vi "manual_display.vi"() -> ()   [LabVIEW 2020]
uses:
  <vilib>/Analysis/1siggen.llb/Ramp Pattern by Samples.vi
  <vilib>/Waveform/WDTOps.llb/WDT Get Waveform Subset DBL.vi
  <vilib>/Analysis/1siggen.llb/Ramp Pattern by Delta.vi
  <vilib>/Analysis/NI_AALBase.lvlib
  <vilib>/Analysis/NI_AALPro.lvlib
panel:
  out "gps-es sebesség\ngrafikon":cluster{timestamp[], "Y":dbl[]}[](graph)
  in  "másolás mód":bool
  in  "gps elcsúsztatás [s]":dbl format="%#_13g"
  out "elemzõ grafikon":T1(graph)
  in  "high cutoff freq":dbl=10.0 format="%#_13g"
  in  "low cutoff freq":dbl=0.05 format="%#_13g"
  out "impulse szum/mean\n(összes csapás az átlagos \ncsapásszámon)":dbl format="%0.2f"
  out "inspected resultant":waveform(dbl)(graph)
  out "Z axis SNR mean":dbl format="%0.2f"
  out "Z axis SNR standard deviation":dbl format="%0.2f"
  out "resultant SNR mean":dbl format="%0.2f"
  out "resultant SNR standard deviation":dbl format="%0.2f"
  out "Y axis SNR mean":dbl format="%0.2f"
  out "Y axis SNR standard deviation":dbl format="%0.2f"
  out "X axis SNR standard deviation":dbl format="%0.2f"
  out "X axis SNR mean":dbl format="%0.2f"
  out "impulse mean":dbl format="%0.2f"
  out "Z axis SNR":cluster{"Ramp Pattern":dbl[], dbl[]}[](graph)
  out "Y axis SNR":cluster{"Ramp Pattern":dbl[], dbl[]}[](graph)
  out "X axis SNR":cluster{"Ramp Pattern":dbl[], dbl[]}[](graph)
  out "resultant SNR":cluster{"Ramp Pattern":dbl[], dbl[]}[](graph)
  in  "felharmonikus N":i32=3
  out "standard deviation of peaks":dbl format="%0.2f"
  out "SNR":dbl
  in  "SNR window width [Hz]":dbl=0.2
  out "impulse  szum":dbl format="%0.2f"
  out "impulse standard deviation":dbl format="%0.2f"
  in  "invert":bool
  out "csapás impulzus":cluster{"Ramp Pattern":dbl[], dbl[]}(graph)
  in  "peak detect width":i32=5 min=3
  in  "avg window size":i32=5
  in  "threshold":dbl=0.25 format="%0.2f"
  out "mean of peaks":dbl format="%0.2f"
  out "csapásszám":cluster{"Ramp Pattern":dbl[], dbl[]}[](graph)
  in  "felbontás [s]":dbl=20.0
  out "Átlag Csapásszám [stroke/m]":dbl
  out "PSD":cluster{"f0":dbl, "df":dbl, "magnitude":dbl[]}[](graph)
  in  "crossing level":dbl
  in  "Cursor reset":bool=TRUE
  out "inspection":cluster{"Y":dbl[], "Y":dbl[]}[](graph)
  in  "Sec":dbl=60.0
  in  "Start Cursor":timestamp
  in  "inspect":bool
  in  "path to binary file":path=path "C:/Users/Lenovo/Desktop/canoe_akti_data"
  in  "stop":bool
  out "inspected section":waveform(dbl)[](graph)
  out "read in data":waveform(dbl)[](graph)
  # "[felbontas]mp-es ablakokkal számított SNR meta adatok"
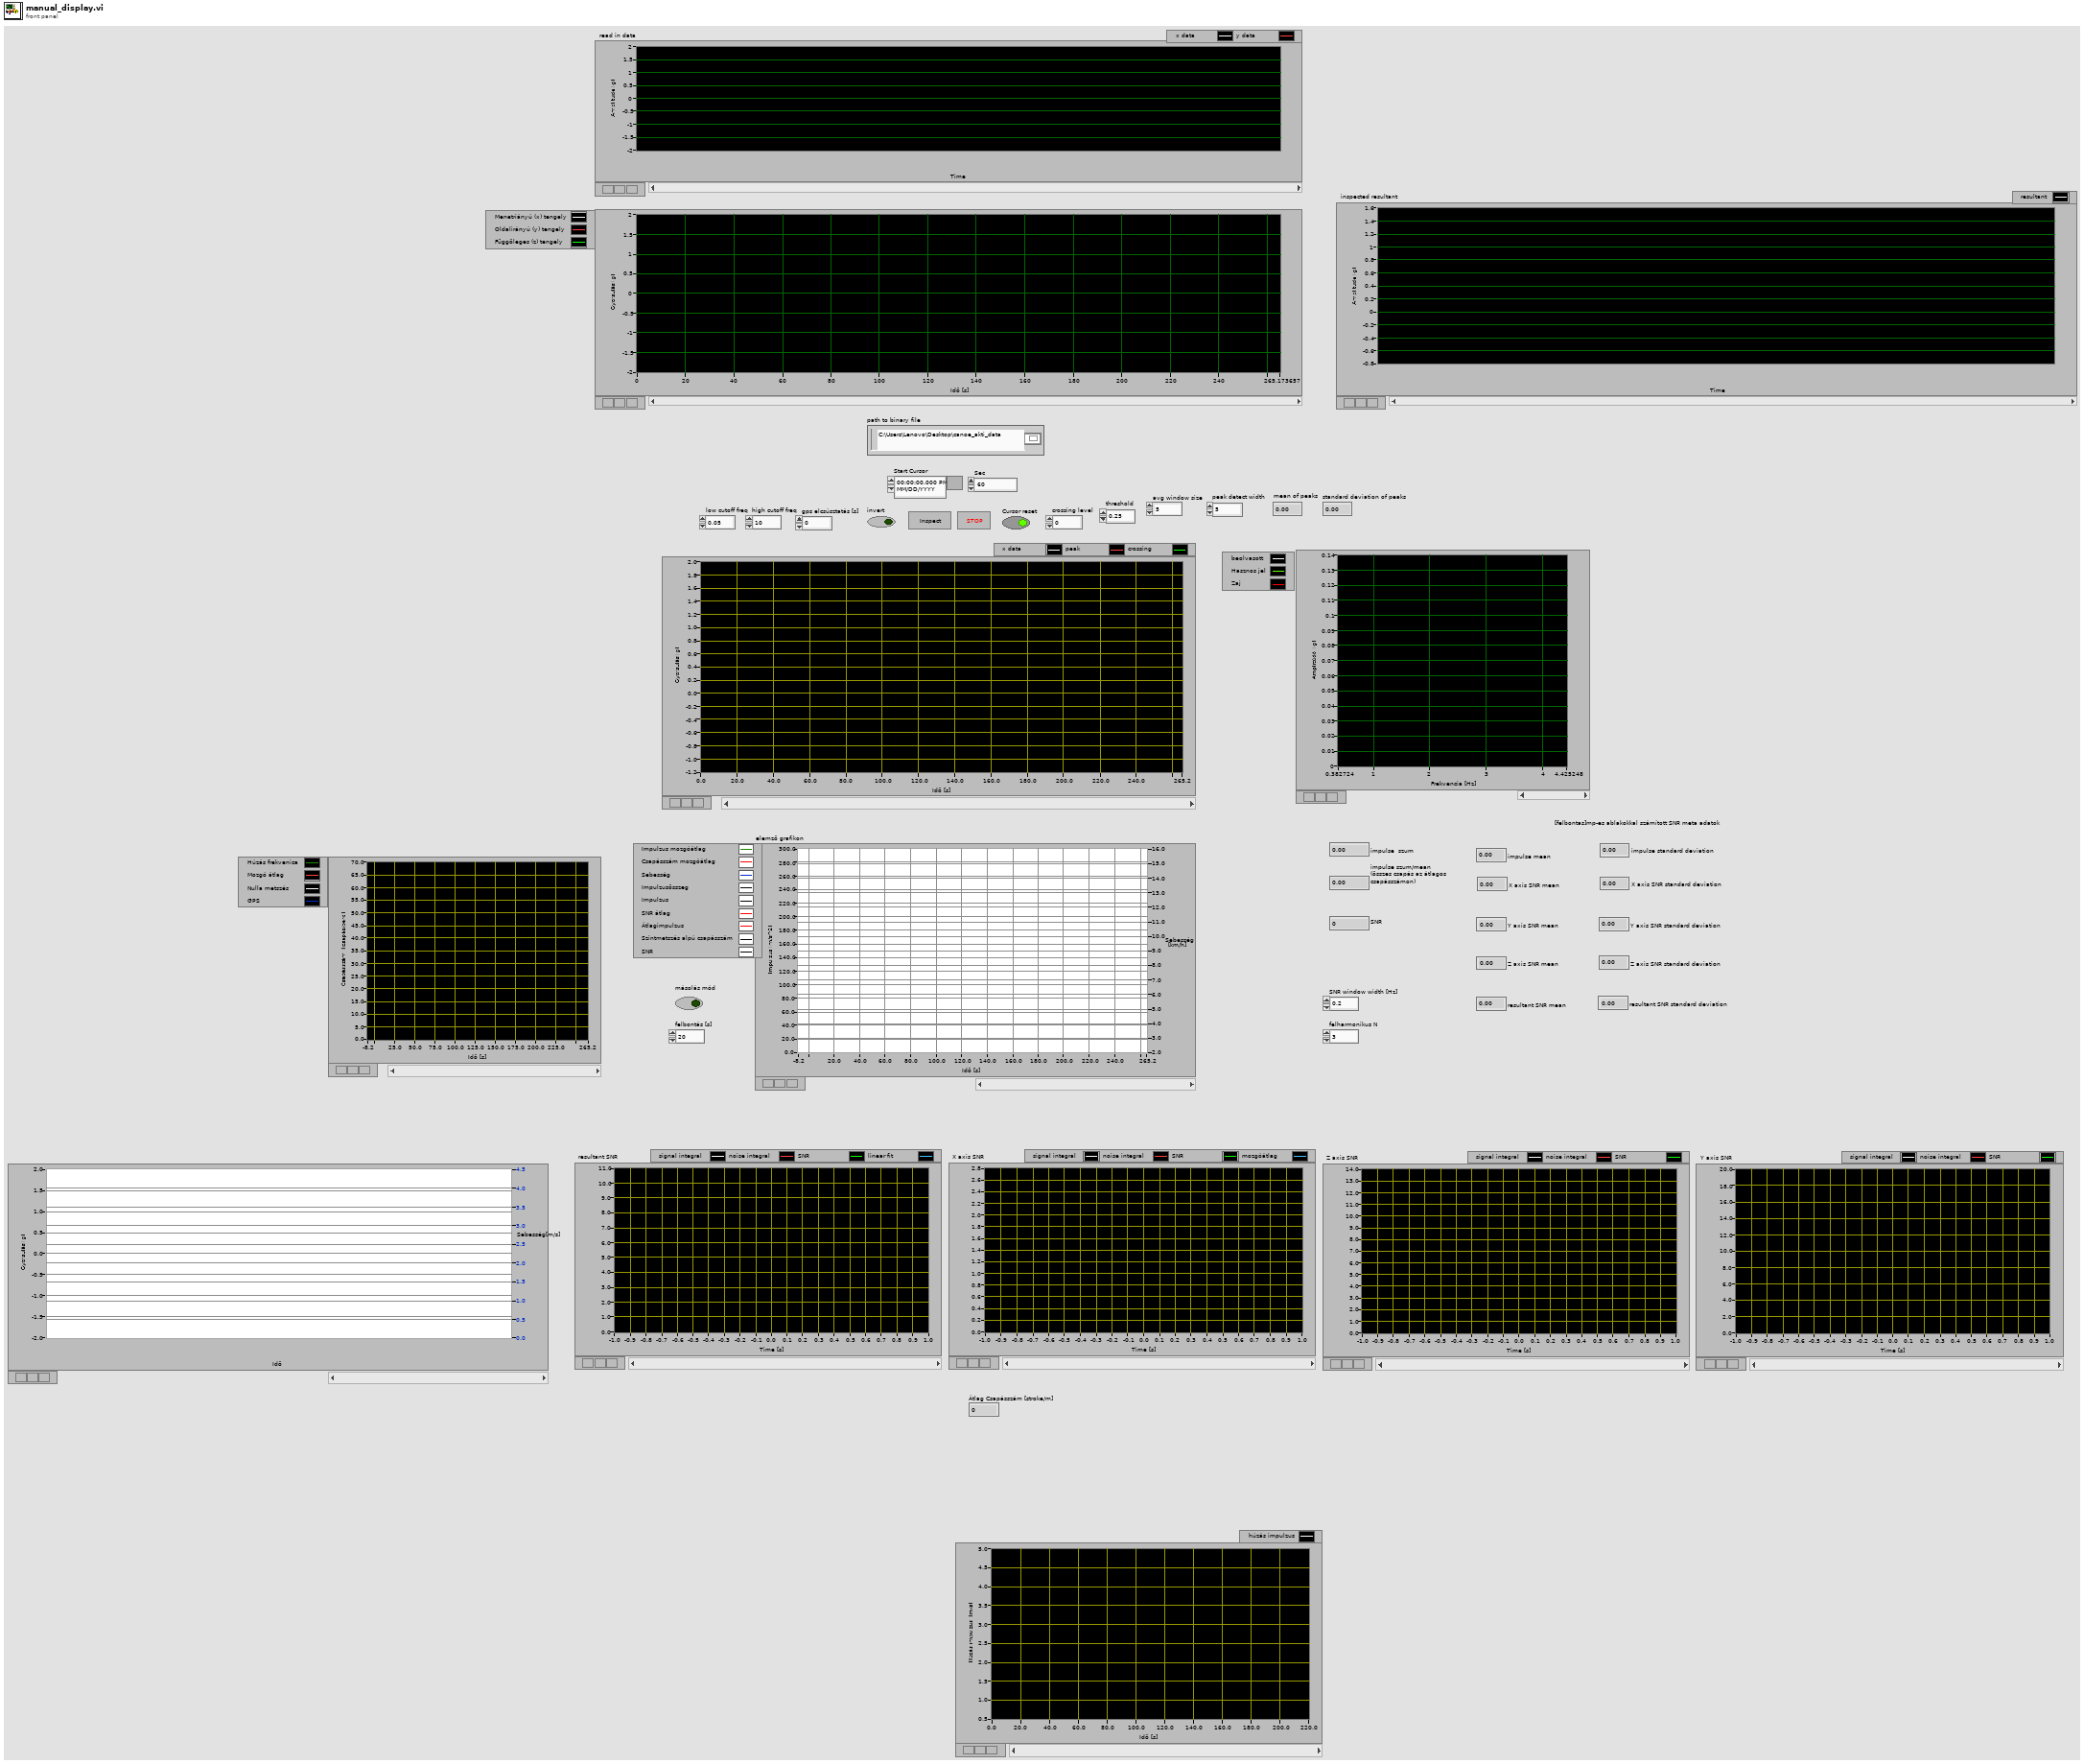
[diagram p1: front panel]
types:
  T1 = cluster{"Ramp Pattern":dbl[], "averaged X":dbl[]}[]
  T2 = typedef "control_all_in_one_package.ctl" = cluster{"memory structure":T3, "actigraph settings":T4, "time informations":T5, "measurement data":T6}
  T3 = typedef "control_memory_structure.ctl" = cluster{"length of metadata [byte]":i32, "length of page [byte]":i32, "length of measurement data on page [byte]":i32, "length of dataset [byte]":i32}
  T4 = typedef "control_measurement_settings.ctl" = cluster{"sampling frequency [Hz]":dbl, "measurement interval [± g]":i32, "high precision?":bool, "number of pages":i32, "rate code":i32, "range code":i32, "id":i32}
  T5 = typedef "control_time_informations.ctl" = cluster{"starting time":timestamp, "ending time":timestamp, "dt[s]":dbl, "sampling rate [Hz]":dbl, "length":dbl}
  T6 = typedef "control_measurement_data.ctl" = cluster{"number of samples per axis":i32, "timestamp array":dbl[], "offset array":dbl[], "x, y, z axis data":waveform(dbl)[], "normalised magnitude of acceleartion vectors":waveform(dbl), "calibration coefficients":T7, "statistics":T8, "battery voltage":waveform(dbl), "magnitude of acceleartion vectors":waveform(dbl)}
  T7 = typedef "control_calibration_coefficients.ctl" = cluster{"Sx":dbl, "Ox":dbl, "Sy":dbl, "Oy":dbl, "Sz":dbl, "Oz":dbl}
  T8 = typedef "control_statistics.ctl" = cluster{"mean of x axis acceleration":dbl, "standard devation of x axis acceleration":dbl, "mean of y axis acceleration":dbl, "standard devation of y axis acceleration":dbl, "mean of z axis acceleration":dbl, "standard devation of z axis acceleration":dbl, "mean of normalised magnitude of acceleration":dbl, "standard devation of normalised magnitude of acceleration":dbl}
  T9 = cluster{"start samples/time":dbl, "duration":dbl, "snr window width [Hz]":dbl, "harmonic N":i32}
  T10 = cluster{"Signal Integral":dbl, "Noise Integral":dbl, "SNR":dbl, "PSD":cluster{"f0":dbl, "df":dbl, "magnitude":dbl[]}[], "Amplitude":dbl, "Frequency":dbl, "Stroke rate [stroke/min]":dbl}
  T11 = cluster{"Ramp Pattern":dbl[], "averaged X":dbl[]}
  T12 = cluster{"Ramp Pattern":dbl[], "stroke rate":dbl[]}
  T13 = cluster{"Ramp Pattern":dbl[], "Best Linear Fit":dbl[]}
  T14 = cluster{"Ramp Pattern":dbl[], "Best Linear Fit":dbl[]}[]
  T15 = cluster{"Ramp Pattern":dbl[], "stroke rate":dbl[]}[]
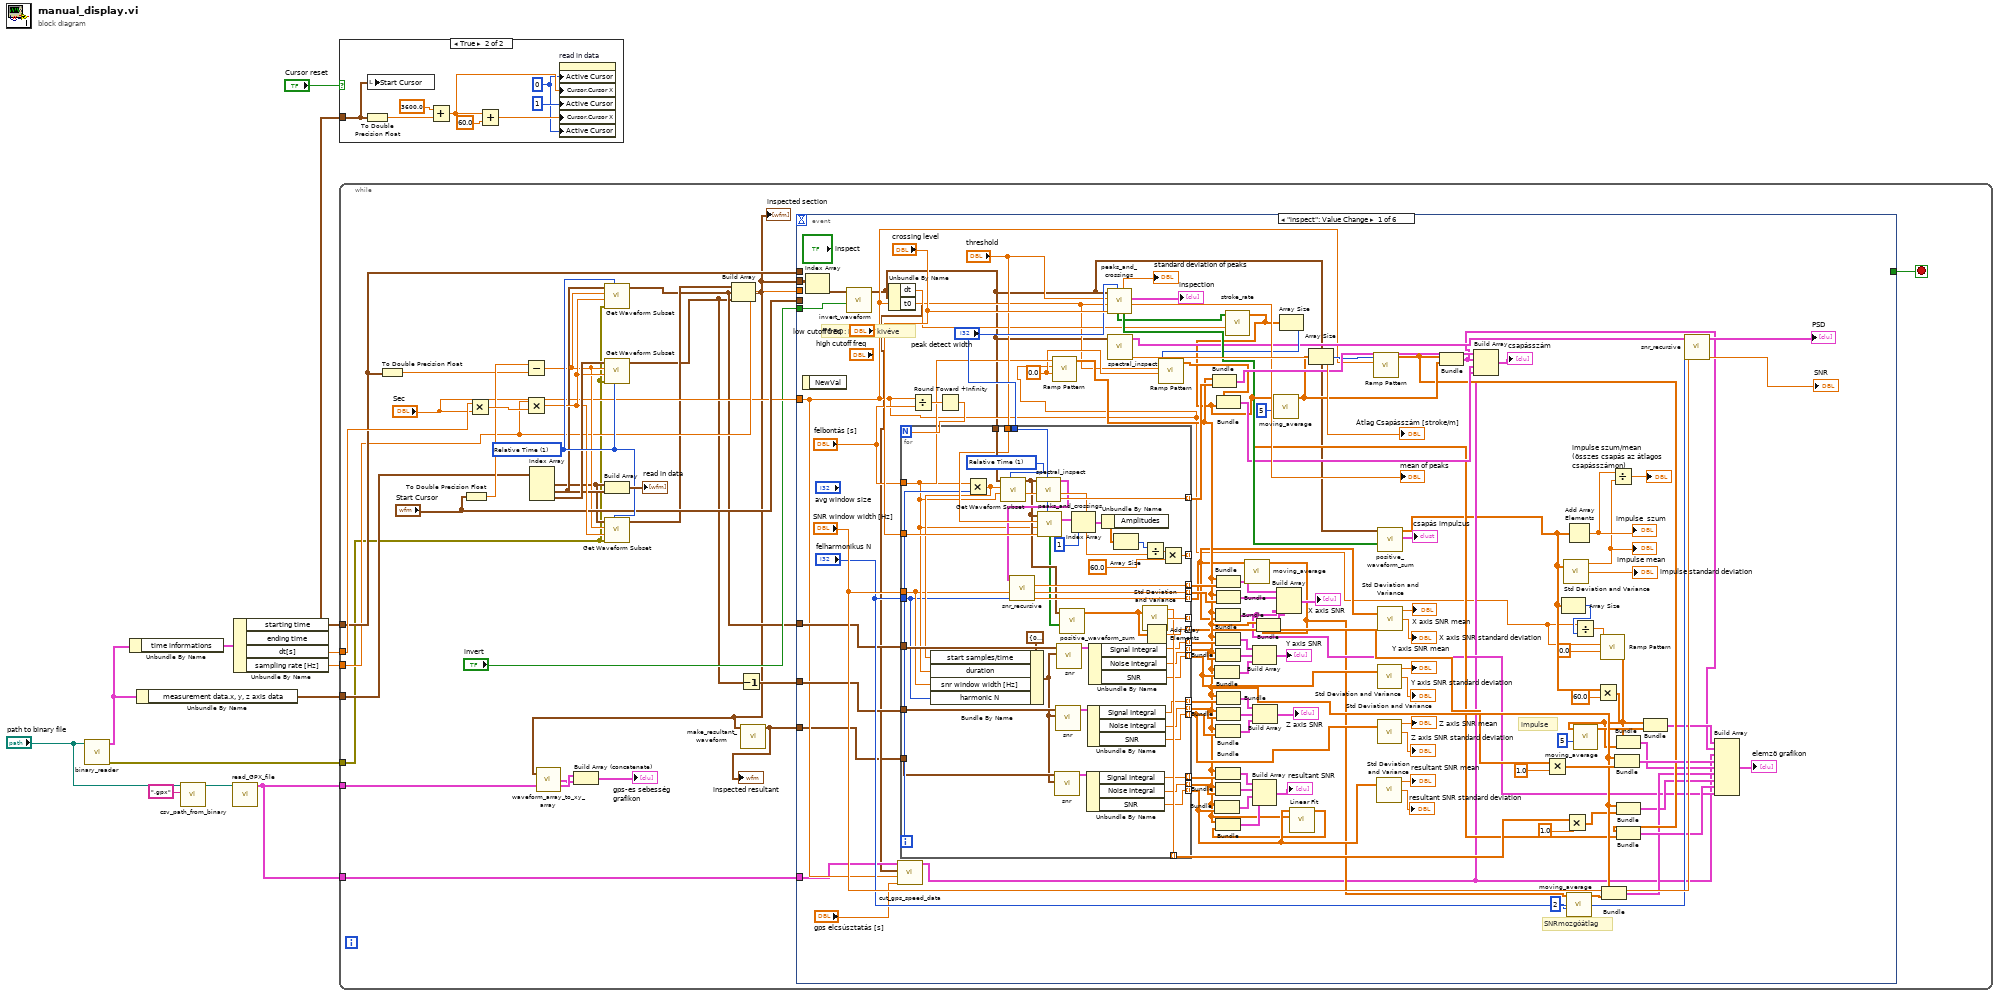
[diagram p0: block diagram]
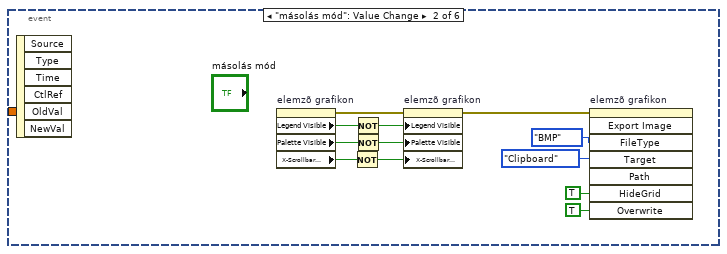
[diagram p3: hidden frame]
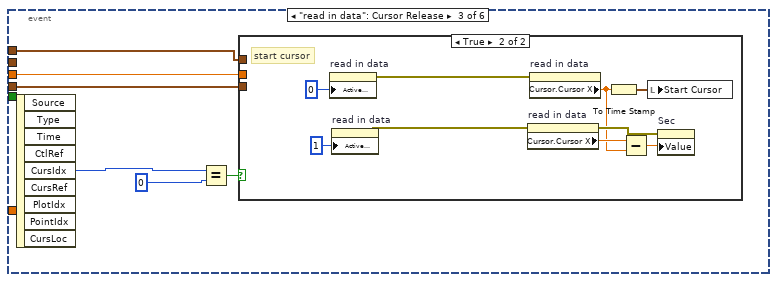
[diagram p4: hidden frame]
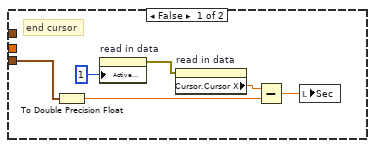
[diagram p5: hidden frame]
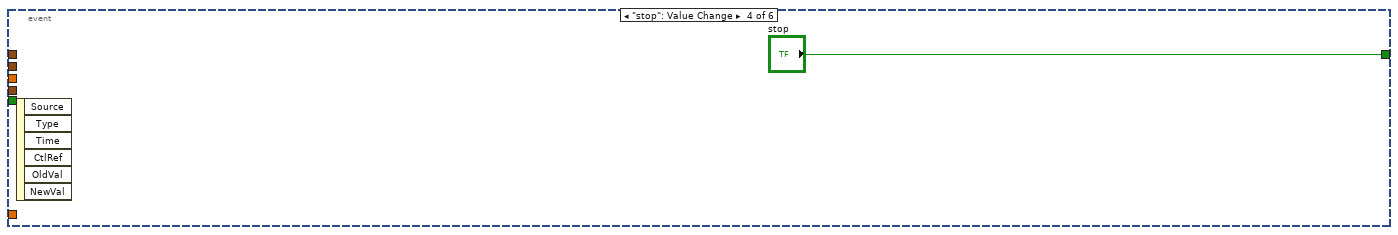
[diagram p6: hidden frame]
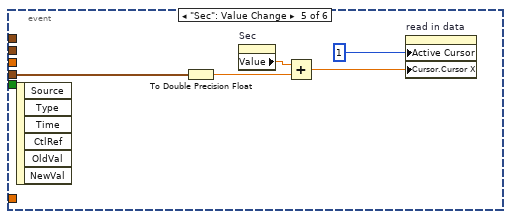
[diagram p7: hidden frame]
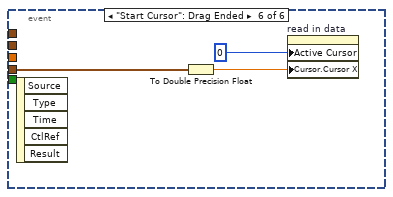
[diagram p8: hidden frame]
diagram:
  n1 = call "binary_reader.vi"("path to binary file"="path to binary file") -> ("error out"=w7:errorcluster, "all in one package"=w2:T2)  [unwired: 7 in, 1 out]
  n2 = Unbundle By Name(w2) -> ("time informations"=w12:T5)
  n3 = Unbundle By Name(w2) -> ("measurement data.x, y, z axis data"=w1:waveform(dbl)[])
  n4 = call "csv_path_from_binary.vi"("extension"=".gpx", "path to binary file"="path to binary file") -> ("path to spec. ext."=w6:path)  [unwired: 9 in]
  n5 = call "read_GPX_file.vi"("GPX File Path"=w6) -> ("XY Speed data"=w3:cluster{timestamp[], dbl[]})  [unwired: 3 in, 3 out]
  n6 = Unbundle By Name(w12) -> ("starting time"=w9:timestamp, "dt[s]"=w10:dbl, "sampling rate [Hz]"=w11:dbl)  [unwired: 1 out]
  n7 = case shown="True" "Cursor reset" {
    tunnel: w9 -> [_ w17]
    frame False {
    }
    frame True {
      w13 = 0
      n8 = To Double Precision Float(number=w17) -> (double precision float=w19:dbl)
      n9 = local write "Start Cursor"(w17) -> ()
      n10 = Add(x=3600.0, y=w19) -> (x+y=w16:dbl)
      n11 = Add(x=w16, y=60.0) -> (x+y=w14:dbl)
      n12 = property on="read in data" class="WFGraph (strict)"("Active Cursor"=w13, "Cursor.Cursor X"=w16, "Active Cursor"=1, "Cursor.Cursor X"=w14, "Active Cursor"=w13) -> ()  [unwired: 2 in, 2 out]
    }
  }
  n13 = while {
    tunnel: w1 -> [w32]
    tunnel: w7 -> [w23]
    tunnel: w11 -> [w36]
    tunnel: w10 -> [w43]
    tunnel: w9 -> [w38]
    tunnel: w3 -> [w25]
    tunnel: w3 -> [w26]
    stop <- w42 stop-if-true
    w48 = u16 1 items=["Samples", "Relative Time"] ("start/duration format")
    n14 = To Double Precision Float(number=w38) -> (double precision float=w39:dbl)
    n15 = To Double Precision Float(number="Start Cursor") -> (double precision float=w40:dbl)
    n16 = Multiply(x=w43, y="Sec") -> (x*y=w45:dbl)
    n17 = Subtract(x=w40, y=w39) -> (x-y=w37:dbl)
    n18 = Multiply(x=w36, y=w45) -> (x*y=w46:dbl)
    n19 = Index Array(array=w32) -> (element #1=w33:waveform(dbl), element #2=w44:waveform(dbl), element #3=w47:waveform(dbl))  [unwired: 3 in]
    n20 = call-poly <vilib>:"Get Waveform Subset.vi"("start/duration format"=w48, "error in (no error)"=w23, "duration"=w46, "start samples/time"=w37, "waveform in"=w44) -> ("waveform out"=w30:waveform(dbl))  [unwired: 1 in, 3 out]
    n21 = call-poly <vilib>:"Get Waveform Subset.vi"("start/duration format"=w48, "error in (no error)"=w23, "duration"=w46, "start samples/time"=w37, "waveform in"=w47) -> ("waveform out"=w28:waveform(dbl))  [unwired: 1 in, 3 out]
    n22 = Build Array(w33, w44) -> (→"read in data":waveform(dbl)[])
    n23 = call-poly <vilib>:"Get Waveform Subset.vi"("start/duration format"=w48, "error in (no error)"=w23, "duration"=w46, "start samples/time"=w37, "waveform in"=w33) -> ("waveform out"=w31:waveform(dbl))  [unwired: 1 in, 3 out]
    n24 = Build Array(w31, w30, w28) -> (w22:waveform(dbl)[])
    "inspected section" <- w22
    n25 = call "waveform_array_to_xy_array.vi"("waveform array"=w22) -> ("XY array"=w21:cluster{timestamp[], "Y":dbl[]}[])  [unwired: 1 in]
    n26 = Build Array (concatenate)(w25, w21) -> (→"gps-es sebesség\ngrafikon":cluster{timestamp[], "Y":dbl[]}[])
    n27 = Decrement(x=w28) -> (x-1=w29:waveform(dbl))
    n28 = call "make_resultant_waveform.vi"("waveform array"=w22) -> ("inspected resultant"=w27:waveform(dbl))  [unwired: 9 in, 1 out]
    "inspected resultant" <- w27
    n29 = event shown="[0] \"inspect\": Value Change" {
      selector: _ -> [_ _ _ _ _ _]
      dyn-events: _ -> [_ _ _ _ _ _]
      timeout: _ -> [_ _ _ _ _ _]
      tunnel: [_ _ _ "stop" _ _] -> w42
      tunnel: w22 -> [w162 _ _ _ _ _]
      tunnel: w38 -> [_ _ w224 _ _ _]
      tunnel: "Start Cursor" -> [_ _ w223 _ w247 w251]
      tunnel: w36 -> [_ _ w222 _ _ _]
      tunnel: "Sec" -> [w54 _ _ _ _ _]
      tunnel: "invert" -> [w148 _ _ _ _ _]
      tunnel: w30 -> [w117 _ _ _ _ _]
      tunnel: w29 -> [w116 _ _ _ _ _]
      tunnel: w27 -> [w51 _ _ _ _ _]
      tunnel: w26 -> [w53 _ _ _ _ _]
      event "inspect": Value Change {
        w146 = 0.0 ("start")
        # "TODO: BWORT kivéve"
        # "impulse"
        # "SNRmozgóátlag"
        n30 = event-data() -> ()  [unwired: 1 in, 1 out]
        n31 = Index Array(array=w162) -> (element=w149:waveform(dbl))  [unwired: 1 in]
        n32 = call "invert_waveform.vi"("invert"=w148, "waveform"=w149) -> ("output waveform"=w50:waveform(dbl))  [unwired: 9 in]
        n33 = Unbundle By Name(w50) -> ("dt"=w95:dbl, "t0"=w52:timestamp)
        n34 = call "cut_gps_speed_data.vi"("gps shift [s]"="gps elcsúsztatás [s]", "Sec"=w54, "Start Time"=w52, "timestamp gps speed data"=w53) -> ("XY gps speed data"=w58:cluster{dbl[], dbl[]})  [unwired: 7 in]
        n35 = Divide(x=w54, y="felbontás [s]") -> (x/y=w159:dbl)
        n36 = Round Toward +Infinity(x=w159) -> (ceil(x): smallest int >= x=w160:dbl)
        n37 = for {
          N: w160 -> [_]
          tunnel: "felbontás [s]" -> [w166]
          tunnel: w50 -> [w209]
          tunnel: [w208] -> w156 mode=indexing
          tunnel: [w200] -> _ mode=indexing
          tunnel: "crossing level" -> [w199]
          tunnel: "peak detect width" -> [w198]
          tunnel: "threshold" -> [w197]
          tunnel: [w181] -> w140 mode=indexing
          tunnel: [w180] -> w139 mode=indexing
          tunnel: [w179] -> w105 mode=indexing
          tunnel: "SNR window width [Hz]" -> [w165]
          tunnel: "felharmonikus N" -> [w164]
          tunnel: [w191] -> w132 mode=indexing
          tunnel: [w193] -> w133 mode=indexing
          tunnel: [w194] -> w64 mode=indexing
          tunnel: [w174] -> w131 mode=indexing
          tunnel: [w173] -> w130 mode=indexing
          tunnel: [w172] -> w107 mode=indexing
          tunnel: [w171] -> w120 mode=indexing
          tunnel: [w170] -> w121 mode=indexing
          tunnel: [w169] -> w94 mode=indexing
          tunnel: w117 -> [w176]
          tunnel: w116 -> [w175]
          tunnel: w51 -> [w183]
          tunnel: [w186] -> _ mode=indexing
          tunnel: [w185] -> w76 mode=indexing
          tunnel: [w184] -> w68 mode=indexing
          i -> [w196]
          w190 = u16 1 items=["Samples", "Relative Time"] ("start/duration format")
          n38 = Multiply(x=w166, y=w196) -> (x*y=w167:dbl)
          n39 = Bundle By Name(cluster=T9 {"start samples/time"=0.0, "duration"=0.0, "snr window width [Hz]"=0.0, "harmonic N"=0} ("snr config"), "start samples/time"=w167, "duration"=w166, "snr window width [Hz]"=w165, "harmonic N"=w164) -> (w163:T9)
          n40 = call-poly <vilib>:"Get Waveform Subset.vi"("start/duration format"=w190, "duration"=w166, "start samples/time"=w167, "waveform in"=w209) -> ("actual duration"=w195:dbl, "waveform out"=w189:waveform(dbl))  [unwired: 2 in, 2 out]
          n41 = call "spectral_inspect.vi"("waveform"=w189) -> ("Csapásszám [stroke/min]"=w208:dbl, "PSD"=w192:cluster{"f0":dbl, "df":dbl, "magnitude":dbl[]})  [unwired: 6 in, 3 out]
          n42 = call "snr_recursive.vi"("felharmonikus N"=w164, "width [Hz]"=w165, "PSD"=w192) -> ("SNR"=w194:dbl, "Noise Integral"=w193:dbl, "Signal Integral"=w191:dbl)  [unwired: 5 in, 1 out]
          n43 = call "peaks_and_crossings.vi"("width"=w198, "crossing level"=w199, "end"=w166, "threshold"=w197, "waveform"=w189) -> ("all in array"=w207:cluster{dbl[], "Amplitudes":dbl[]}[], "plus-minus crossing?"=w188:bool[])  [unwired: 5 out]
          n44 = call "snr.vi"("snr config"=w163, "waveform"=w183) -> ("SNR data"=w182:T10)  [unwired: 8 in, 1 out]
          n45 = call "snr.vi"("snr config"=w163, "waveform"=w175) -> ("SNR data"=w178:T10)  [unwired: 8 in, 1 out]
          n46 = call "snr.vi"("snr config"=w163, "waveform"=w176) -> ("SNR data"=w177:T10)  [unwired: 8 in, 1 out]
          n47 = call "positive_waveform_sum.vi"("plus-minus"=w188, "read in data"=w189) -> ("Integral X"=w187:dbl[])  [unwired: 8 in, 1 out]
          n48 = Index Array(array=w207, index=1) -> (element=w205:cluster{dbl[], "Amplitudes":dbl[]})
          n49 = Unbundle By Name(w182) -> ("Signal Integral"=w181:dbl, "Noise Integral"=w180:dbl, "SNR"=w179:dbl)
          n50 = Unbundle By Name(w178) -> ("Signal Integral"=w171:dbl, "Noise Integral"=w170:dbl, "SNR"=w169:dbl)
          n51 = Unbundle By Name(w177) -> ("Signal Integral"=w174:dbl, "Noise Integral"=w173:dbl, "SNR"=w172:dbl)
          n52 = Unbundle By Name(w205) -> ("Amplitudes"=w204:dbl[])
          n53 = Array Size(array=w204) -> (size(s)=w203:i32)
          n54 = Divide(x=w203, y=w195) -> (x/y=w202:dbl)
          n55 = call <vilib>:"Std Deviation and Variance.vi"("X"=w187) -> ("mean"=w184:dbl, "standard deviation"=w186:dbl)  [unwired: 1 in, 1 out]
          n56 = Add Array Elements(numeric array=w187) -> (sum=w185:dbl)
          n57 = Multiply(x=w202, y=60.0) -> (x*y=w200:dbl)
        }
        n58 = call-poly <vilib>:"Ramp Pattern.vi"("start"=w146, "end"=w54, "delta"="felbontás [s]") -> ("Ramp Pattern"=w80:dbl[])  [unwired: 6 in, 2 out]
        n59 = call "peaks_and_crossings.vi"("width"="peak detect width", "crossing level"="crossing level", "end"=w54, "threshold"="threshold", "waveform"=w50) -> ("mean of peaks"=→"mean of peaks":dbl, "all in array"=→"inspection":cluster{dbl[], "Amplitudes":dbl[]}[], "plus-minus crossing?"=w150:bool[], "standard deviation of peaks"=→"standard deviation of peaks":dbl, "minus-plus crossing?"=w147:bool[])  [unwired: 2 out]
        n60 = call "spectral_inspect.vi"("waveform"=w50) -> ("Csapásszám [stroke/min]"=→"Átlag Csapásszám [stroke/m]":dbl, "PSD"=w141:cluster{"f0":dbl, "df":dbl, "magnitude":dbl[]})  [unwired: 6 in, 3 out]
        n61 = Bundle("Ramp Pattern"=w80, w156) -> (w158:cluster{"Ramp Pattern":dbl[], dbl[]})  [unwired: 1 in]
        n62 = Bundle("Ramp Pattern"=w80, w107) -> (w127:cluster{"Ramp Pattern":dbl[], dbl[]})  [unwired: 1 in]
        n63 = Bundle("Ramp Pattern"=w80, w105) -> (w136:cluster{"Ramp Pattern":dbl[], dbl[]})  [unwired: 1 in]
        n64 = Bundle("Ramp Pattern"=w80, w64) -> (w60:cluster{"Ramp Pattern":dbl[], dbl[]})  [unwired: 1 in]
        n65 = Bundle("Ramp Pattern"=w80, w131) -> (w129:cluster{"Ramp Pattern":dbl[], dbl[]})  [unwired: 1 in]
        n66 = Bundle("Ramp Pattern"=w80, w130) -> (w128:cluster{"Ramp Pattern":dbl[], dbl[]})  [unwired: 1 in]
        n67 = Bundle("Ramp Pattern"=w80, w94) -> (w124:cluster{"Ramp Pattern":dbl[], dbl[]})  [unwired: 1 in]
        n68 = Bundle("Ramp Pattern"=w80, w140) -> (w138:cluster{"Ramp Pattern":dbl[], dbl[]})  [unwired: 1 in]
        n69 = Bundle("Ramp Pattern"=w80, w139) -> (w137:cluster{"Ramp Pattern":dbl[], dbl[]})  [unwired: 1 in]
        n70 = Bundle("Ramp Pattern"=w80, w132) -> (w90:cluster{"Ramp Pattern":dbl[], dbl[]})  [unwired: 1 in]
        n71 = Bundle("Ramp Pattern"=w80, w133) -> (w134:cluster{"Ramp Pattern":dbl[], dbl[]})  [unwired: 1 in]
        n72 = Bundle("Ramp Pattern"=w80, w120) -> (w122:cluster{"Ramp Pattern":dbl[], dbl[]})  [unwired: 1 in]
        n73 = Bundle("Ramp Pattern"=w80, w121) -> (w123:cluster{"Ramp Pattern":dbl[], dbl[]})  [unwired: 1 in]
        n74 = call "stroke_rate.vi"("dt"=w95, "minus-plus"=w147) -> ("stroke rate"=w67:dbl[])  [unwired: 9 in]
        n75 = call "moving_average.vi"("X"=w64) -> ("averaged X"=w59:dbl[])  [unwired: 10 in]
        n76 = Build Array(w129, w128, w127) -> (→"Y axis SNR":cluster{"Ramp Pattern":dbl[], dbl[]}[])
        n77 = Build Array(w122, w123, w124) -> (→"Z axis SNR":cluster{"Ramp Pattern":dbl[], dbl[]}[])
        n78 = Bundle("Ramp Pattern"=w80, "averaged X"=w59) -> (w65:T11)  [unwired: 1 in]
        n79 = call "moving_average.vi"("window size"=5, "X"=w67) -> ("averaged X"=w98:dbl[])  [unwired: 9 in]
        n80 = Build Array(w90, w134, w60, w65) -> (→"X axis SNR":T1)
        n81 = Array Size(array=w67) -> (size(s)=w145:i32)
        n82 = call-poly <vilib>:"Ramp Pattern.vi"("start"=w146, "end"=w54, "samples"=w145) -> ("Ramp Pattern"=w97:dbl[])  [unwired: 7 in, 1 out]
        n83 = Bundle("Ramp Pattern"=w97, "stroke rate"=w67) -> (w96:T12)  [unwired: 1 in]
        n84 = call <vilib>:"Linear Fit.vi"("Y"=w105, "X"=w80) -> ("Best Linear Fit"=w103:dbl[])  [unwired: 9 in, 4 out]
        n85 = Bundle("Ramp Pattern"=w80, "Best Linear Fit"=w103) -> (w104:T13)  [unwired: 1 in]
        n86 = Build Array(w138, w137, w136, w104) -> (→"resultant SNR":T14)
        n87 = Array Size(array=w98) -> (size(s)=w66:i32)
        n88 = call-poly <vilib>:"Ramp Pattern.vi"("end"=w54, "samples"=w66) -> ("Ramp Pattern"=w84:dbl[])  [unwired: 8 in, 1 out]
        n89 = call <vilib>:"Std Deviation and Variance.vi"("X"=w105) -> ("mean"=→"resultant SNR mean":dbl, "standard deviation"=→"resultant SNR standard deviation":dbl)  [unwired: 1 in, 1 out]
        n90 = call <vilib>:"Std Deviation and Variance.vi"("X"=w107) -> ("mean"=→"Y axis SNR mean":dbl, "standard deviation"=→"Y axis SNR standard deviation":dbl)  [unwired: 1 in, 1 out]
        n91 = call <vilib>:"Std Deviation and Variance.vi"("X"=w94) -> ("mean"=→"Z axis SNR mean":dbl, "standard deviation"=→"Z axis SNR standard deviation":dbl)  [unwired: 1 in, 1 out]
        n92 = call "positive_waveform_sum.vi"("plus-minus"=w150, "read in data"=w50) -> ("csapás impulzus"=→"csapás impulzus":cluster{"Ramp Pattern":dbl[], dbl[]}, "Integral X"=w56:dbl[])  [unwired: 8 in]
        n93 = call <vilib>:"Std Deviation and Variance.vi"("X"=w64) -> ("mean"=→"X axis SNR mean":dbl, "standard deviation"=→"X axis SNR standard deviation":dbl)  [unwired: 1 in, 1 out]
        n94 = Bundle("Ramp Pattern"=w84, "averaged X"=w98) -> (w73:T11)  [unwired: 1 in]
        n95 = Build Array(w158, w73, w96, w58) -> (→"csapásszám":T15)
        n96 = Multiply(x=w76, y=1.0) -> (x*y=w81:dbl[])
        n97 = Array Size(array=w56) -> (size(s)=w86:i32)
        n98 = call <vilib>:"Std Deviation and Variance.vi"("X"=w56) -> ("mean"=w100:dbl, "standard deviation"=→"impulse standard deviation":dbl)  [unwired: 1 in, 1 out]
        "impulse mean" <- w100
        n99 = Multiply(x=w68, y=1.0) -> (x*y=w63:dbl[])
        n100 = Add Array Elements(numeric array=w56) -> (sum=w101:dbl)
        "impulse  szum" <- w101
        n101 = call "moving_average.vi"("window size"=2, "X"=w59) -> ("averaged X"=w83:dbl[])  [unwired: 9 in]
        n102 = Divide(x=w54, y=w86) -> (x/y=w87:dbl)
        n103 = Multiply(x=w56, y=60.0) -> (x*y=w70:dbl[])
        n104 = call "moving_average.vi"("window size"=5, "X"=w70) -> ("averaged X"=w79:dbl[])  [unwired: 9 in]
        n105 = call-poly <vilib>:"Ramp Pattern.vi"("start"=0.0, "end"=w54, "delta"=w87) -> ("Ramp Pattern"=w78:dbl[])  [unwired: 6 in, 2 out]
        n106 = Bundle("Ramp Pattern"=w80, "averaged X"=w83) -> (w62:T11)  [unwired: 1 in]
        n107 = Divide(x=w101, y=w100) -> (x/y=→"impulse szum/mean\n(összes csapás az átlagos \ncsapásszámon)":dbl)
        n108 = Bundle("Ramp Pattern"=w80, w81) -> (w89:cluster{"Ramp Pattern":dbl[], dbl[]})  [unwired: 1 in]
        n109 = Bundle("Ramp Pattern"=w78, w70) -> (w75:cluster{"Ramp Pattern":dbl[], dbl[]})  [unwired: 1 in]
        n110 = Bundle("Ramp Pattern"=w80, w63) -> (w61:cluster{"Ramp Pattern":dbl[], dbl[]})  [unwired: 1 in]
        n111 = Bundle("Ramp Pattern"=w84, "stroke rate"=w67) -> (w72:T12)  [unwired: 1 in]
        n112 = Bundle("Ramp Pattern"=w78, "averaged X"=w79) -> (w74:T11)  [unwired: 1 in]
        n113 = call "snr_recursive.vi"("felharmonikus N"="felharmonikus N", "width [Hz]"="SNR window width [Hz]", "PSD"=w141) -> ("SNR"=→"SNR":dbl, "PSD"=→"PSD":cluster{"f0":dbl, "df":dbl, "magnitude":dbl[]}[])  [unwired: 5 in, 2 out]
        n114 = Build Array(w74, w73, w58, w89, w75, w62, w61, w72, w60) -> (→"elemzõ grafikon":T15)
      }
      event "másolás mód": Value Change {
        n115 = event-data() -> ()  [unwired: 1 in, 6 out]
        n116 = property on="elemzõ grafikon" class="XYGraph (strict)"() -> (error out=w216:errorcluster, "Legend Visible"=w215:bool, "Palette Visible"=w212:bool, "X-Scrollbar Visible"=w214:bool)  [unwired: 2 in, 1 out]
        n117 = Not(x=w214) -> (.not. x?=w210:bool)
        n118 = Not(x=w215) -> (.not. x?=w213:bool)
        n119 = Not(x=w212) -> (.not. x?=w211:bool)
        n120 = property on="elemzõ grafikon" class="XYGraph (strict)"(error in=w216, "Legend Visible"=w213, "Palette Visible"=w211, "X-Scrollbar Visible"=w210) -> (error out=w217:errorcluster)  [unwired: 1 in, 1 out]
        n121 = invoke on="elemzõ grafikon" class="XYGraph (strict)" method="Export Image"(error in=w217, "FileType"=enum32{"BMP", "EPS", "EMF", "PICT"}."BMP" ("File Type"), "Target"=enum32{"File", "Clipboard"}."Clipboard", "HideGrid"=TRUE ("Hide Grid"), "Overwrite"=TRUE ("Always Overwrite")) -> ()  [unwired: 3 in, 8 out]
      }
      event "read in data": Cursor Release {
        n122 = event-data() -> ("CursIdx"=w227:i32)  [unwired: 1 in, 8 out]
        n123 = Equal?(x=w227, y=0) -> (x = y?=w225:bool)
        n124 = case shown="True" w225 {
          tunnel: w224 -> [_ _]
          tunnel: w223 -> [w230 _]
          tunnel: w222 -> [_ _]
          frame False {
            # "end cursor"
            n125 = To Double Precision Float(number=w230) -> (double precision float=w231:dbl)
            n126 = property on="read in data" class="WFGraph (strict)"("Active Cursor"=1) -> (error out=w229:errorcluster)  [unwired: 2 in, 1 out]
            n127 = property on="read in data" class="WFGraph (strict)"(error in=w229) -> ("Cursor.Cursor X"=w232:dbl)  [unwired: 1 in, 2 out]
            n128 = Subtract(x=w232, y=w231) -> (x-y=w228:dbl)
            n129 = local write "Sec"(w228) -> ()
          }
          frame True {
            # "start cursor"
            n130 = property on="read in data" class="WFGraph (strict)"("Active Cursor"=0) -> (error out=w240:errorcluster)  [unwired: 2 in, 1 out]
            n131 = property on="read in data" class="WFGraph (strict)"("Active Cursor"=u32 1) -> (error out=w238:errorcluster)  [unwired: 2 in, 1 out]
            n132 = property on="read in data" class="WFGraph (strict)"(error in=w238) -> (error out=w237:errorcluster, "Cursor.Cursor X"=w235:dbl)  [unwired: 1 in, 1 out]
            n133 = property on="read in data" class="WFGraph (strict)"(error in=w240) -> ("Cursor.Cursor X"=w234:dbl)  [unwired: 1 in, 2 out]
            n134 = To Time Stamp(1:w234) -> (0:w242:timestamp)
            n135 = Subtract(x=w235, y=w234) -> (x-y=w236:dbl)
            n136 = local write "Start Cursor"(w242) -> ()
            n137 = property on="Sec" class="DigNum (strict)"(error in=w237, "Value"=w236) -> ()  [unwired: 1 in, 2 out]
          }
        }
      }
      event "stop": Value Change {
        n138 = event-data() -> ()  [unwired: 1 in, 6 out]
      }
      event "Sec": Value Change {
        n139 = event-data() -> ()  [unwired: 1 in, 6 out]
        n140 = To Double Precision Float(number=w247) -> (double precision float=w246:dbl)
        n141 = property on="Sec" class="DigNum (strict)"() -> ("Value"=w248:dbl)  [unwired: 2 in, 2 out]
        n142 = Add(x=w248, y=w246) -> (x+y=w245:dbl)
        n143 = property on="read in data" class="WFGraph (strict)"("Active Cursor"=u32 1, "Cursor.Cursor X"=w245) -> ()  [unwired: 2 in, 2 out]
      }
      event "Start Cursor": Drag Ended {
        n144 = event-data() -> ()  [unwired: 1 in, 5 out]
        n145 = To Double Precision Float(number=w251) -> (double precision float=w249:dbl)
        n146 = property on="read in data" class="WFGraph (strict)"("Active Cursor"=u32 0, "Cursor.Cursor X"=w249) -> ()  [unwired: 2 in, 2 out]
      }
    }
  }
